vi "Get LabVIEW Version Year.vi"() -> (0 "LabVIEW Version Year":string)   [LabVIEW 2022 SP3]
doc: "This VI returns the LabVIEW Version Year.\n\nFor example when called from:\nLabVIEW 2016 -> returns \"2016\"\nLabVIEW 2018 -> returns \"2018\"\nLabVIEW 2020 -> returns \"2020\"\nLabVIEW 2021 -> returns \"2021\"\nLabVIEW 2022 -> returns \"2022\""
panel:
  # "Development\nControls or indicators that are useful for development or testing, but which are not outputs of the VI."
  # "Input\nInputs to the VI"
  # "Output\nOutputs of the VI"
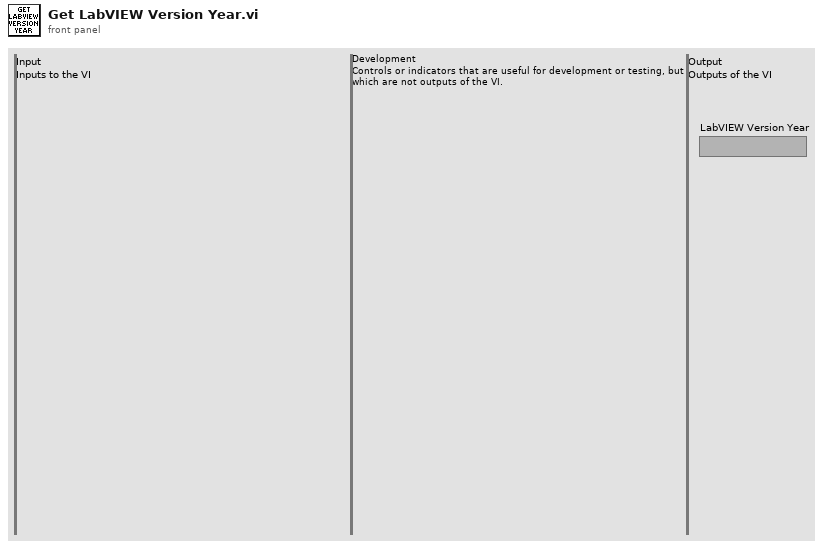
[diagram p1: front panel]
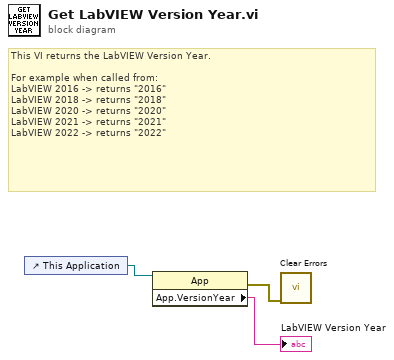
[diagram p0: block diagram]
diagram:
  # "This VI returns the LabVIEW Version Year.\n\nFor example when called from:\nLabVIEW 2016 -> returns \"2016\"\nLabVIEW 2018 -> returns \"2018\"\nLabVIEW 2020 -> returns \"2020\"\nLabVIEW 2021 -> returns \"2021\"\nLabVIEW 2022 -> returns \"2022\""
  n1 = control-ref of="This Application"() -> (w3:refnum<vi>)
  n2 = property class="App"(reference=w3) -> (error out=w1:errorcluster, "App.VersionYear"=→"LabVIEW Version Year":string)  [unwired: 1 in, 1 out]
  n3 = call <vilib>:"Clear Errors.vi"("error in (no error)"=w1) -> ()  [unwired: 5 in, 2 out]
